vi "Strings.vi"() -> ()   [LabVIEW 2020]
uses:
  c5c4e588-2033-429a-969a-39fff3336798.vi
  685e62f0-2af9-4f10-a6a8-997b7a51fd57.vi
  4d49a5eb-9da4-4064-b713-16a5944244b5.vi
panel:
  out "length 3":i32
  out "length 2":i32
  out "x = y? 2":bool[](array[boolean])
  out "length":i32
  out "x = y?":bool
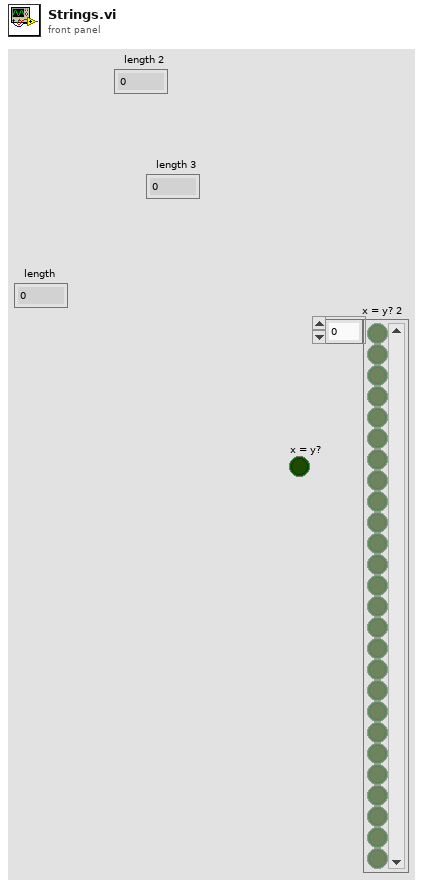
[diagram p1: front panel]
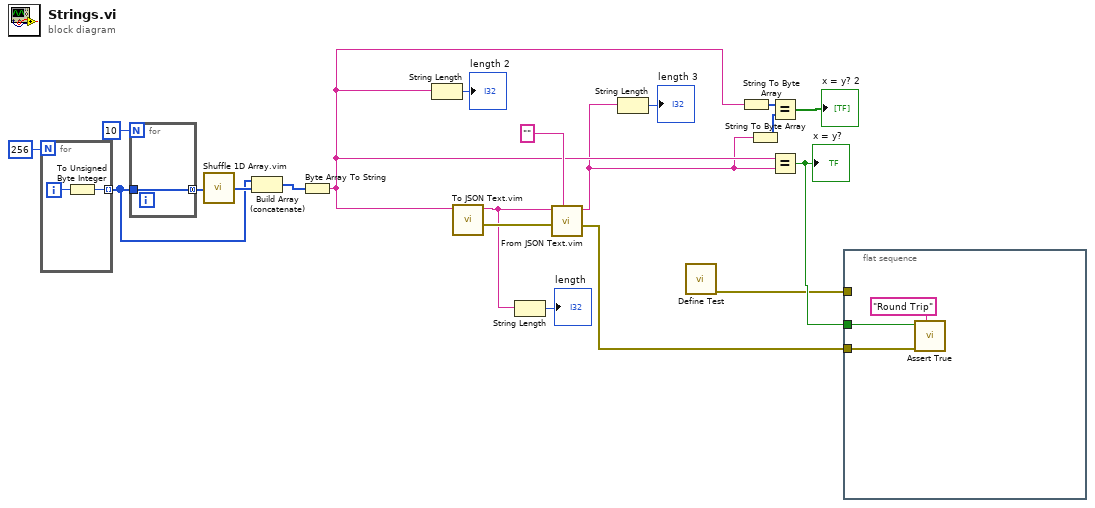
[diagram p0: block diagram]
diagram:
  n1 = for {
    N: 256 -> [_]
    tunnel: [w21] -> w10 mode=indexing
    i -> [w22]
    n2 = To Unsigned Byte Integer(number=w22) -> (unsigned 8bit integer=w21:u8)
  }
  n3 = for {
    N: 10 -> [_]
    tunnel: w10 -> [w23]
    tunnel: [w23] -> w11 mode=concatenating
  }
  n4 = call "Shuffle 1D Array.vim"("array"=w11) -> ("shuffled array"=w14:u8[])  [unwired: 4 in]
  n5 = Build Array (concatenate)(w10, w14) -> (w12:u8[])
  n6 = Byte Array To String(unsigned byte array=w12) -> (string=w3:string)
  n7 = String Length(string=w3) -> (length=→"length 2":i32)
  n8 = call "To JSON Text.vim"("Anything"=w3) -> ("error out"=w17:errorcluster, "<JSON>"=w8:string)  [unwired: 9 in]
  n9 = String Length(string=w8) -> (length=→"length":i32)
  n10 = call "From JSON Text.vim"("Data Type and Default Value"="", "error in (no error)"=w17, "JSON"=w8) -> ("error out"=w15:errorcluster, "Data out"=w1:string)  [unwired: 7 in]
  n11 = String Length(string=w1) -> (length=→"length 3":i32)
  n12 = call <vilib>:"Define Test.vi"() -> ("error out"=w16:errorcluster)  [unwired: 11 in]
  n13 = String To Byte Array(string=w3) -> (unsigned byte array=w6:u8[])
  n14 = String To Byte Array(string=w1) -> (unsigned byte array=w5:u8[])
  n15 = Equal?(x=w6, y=w5) -> (x = y?=→"x = y? 2":bool[])
  n16 = Equal?(x=w3, y=w1) -> (x = y?=w19:bool)
  "x = y?" <- w19
  n17 = flat-sequence {
    tunnel: w19 -> [w25]
    tunnel: w16 -> [_]
    tunnel: w15 -> [w24]
    frame #0 {
      n18 = call <vilib>:"Assert True.vi"("Label"="Round Trip", "error in (no error)"=w24, "True?"=w25) -> ()  [unwired: 8 in, 1 out]
    }
  }
